vi "PollEngine.Main.vi"(8 "error in (no error)":errorcluster, 11 "Parameters":T1 {"Settings"."Data Refs"."Write Refs" format="%.0x"; "Settings"."Data Refs"."Read Refs" format="%.0x"; "Settings"."Write Locations"."DataType" items=["Boolean"=1, "SByte"=2, "Byte"=3, "Int16"=4, "UInt16"=5, "Int32"=6, "UInt32"=7, "Int64"=8, "UInt64"=9, "Float"=10, "Double"=11, "String"=12, "DateTime"=13, "ByteString"=15, "Array of Boolean"=101, "Array of SByte"=102, "Array of Byte"=103, "Array of Int16"=104, "Array of UInt16"=105, "Array of Int32"=106, "Array of UInt32"=107, "Array of Int64"=108, "Array of UInt64"=109, "Array of Float"=110, "Array of Double"=111, "Array of String"=112, "Array of DateTime"=113, "Array of ByteString"=115]; "Settings"."StatusRefs"."Chan Refs" format="%.0x"}) -> ()   [LabVIEW 2013, in "OPC UA Client Engine.lvlib"]
uses:
  OPC UA Client Engine.lvlib
  Types/PollEngine.Parameters.ctl
  Shared/Compiled.Settings.ctl
  Shared/Connection.Properties.ctl
  Shared/PollEngine.Settings.ctl
  <vilib>/NI Veristand/Custom Device API/Data Reference.ctl
  Shared/WriteData.Info.ctl
  Shared/ReadWriteRefs.ctl
  Stop FG/Stop Global Commands.ctl
  Shared/DataRefs.Location.ctl
  <vilib>/OPCUA/client/Write Bool.vi
  <vilib>/OPCUA/client/Write SByte.vi
  <vilib>/OPCUA/client/Write Byte.vi
  <vilib>/OPCUA/client/Write Int16.vi
  <vilib>/OPCUA/client/Write UInt16.vi
  <vilib>/OPCUA/client/Write Int32.vi
  <vilib>/OPCUA/client/Write UInt32.vi
  <vilib>/OPCUA/client/Write Int64.vi
  <vilib>/OPCUA/client/Write UInt64.vi
  <vilib>/OPCUA/client/Write Float.vi
  <vilib>/OPCUA/client/Write Double.vi
  <vilib>/OPCUA/client/Write DateTime.vi
  <vilib>/OPCUA/client/Write Bool Array.vi
  <vilib>/OPCUA/client/Write SByte Array.vi
  <vilib>/OPCUA/client/Write Byte Array.vi
  <vilib>/OPCUA/client/Write Int16 Array.vi
  <vilib>/OPCUA/client/Write UInt16 Array.vi
  <vilib>/OPCUA/client/Write Int32 Array.vi
  <vilib>/OPCUA/client/Write UInt32 Array.vi
  <vilib>/OPCUA/client/Write Int64 Array.vi
  <vilib>/OPCUA/client/Write UInt64 Array.vi
  <vilib>/OPCUA/client/Write Float Array.vi
  <vilib>/OPCUA/client/Write Double Array.vi
  <vilib>/OPCUA/client/Write DateTime Array.vi
  <vilib>/OPCUA/NI OPC UA Client.lvlib
  Stop FG/Stop FG.lvlib
  Error Handling API/Error Handling API.lvlib
  Shared/OPC UA Client Shared.lvlib
  <vilib>/NI Veristand/Custom Device API/Custom Device API.lvlib
panel:
  in  "Parent":string
  out "Read Code":i32
  out "Write Code":i32
  out "Read Table":variant
  out "Write Table":variant
  out "error out":errorcluster
  in  "stop":bool
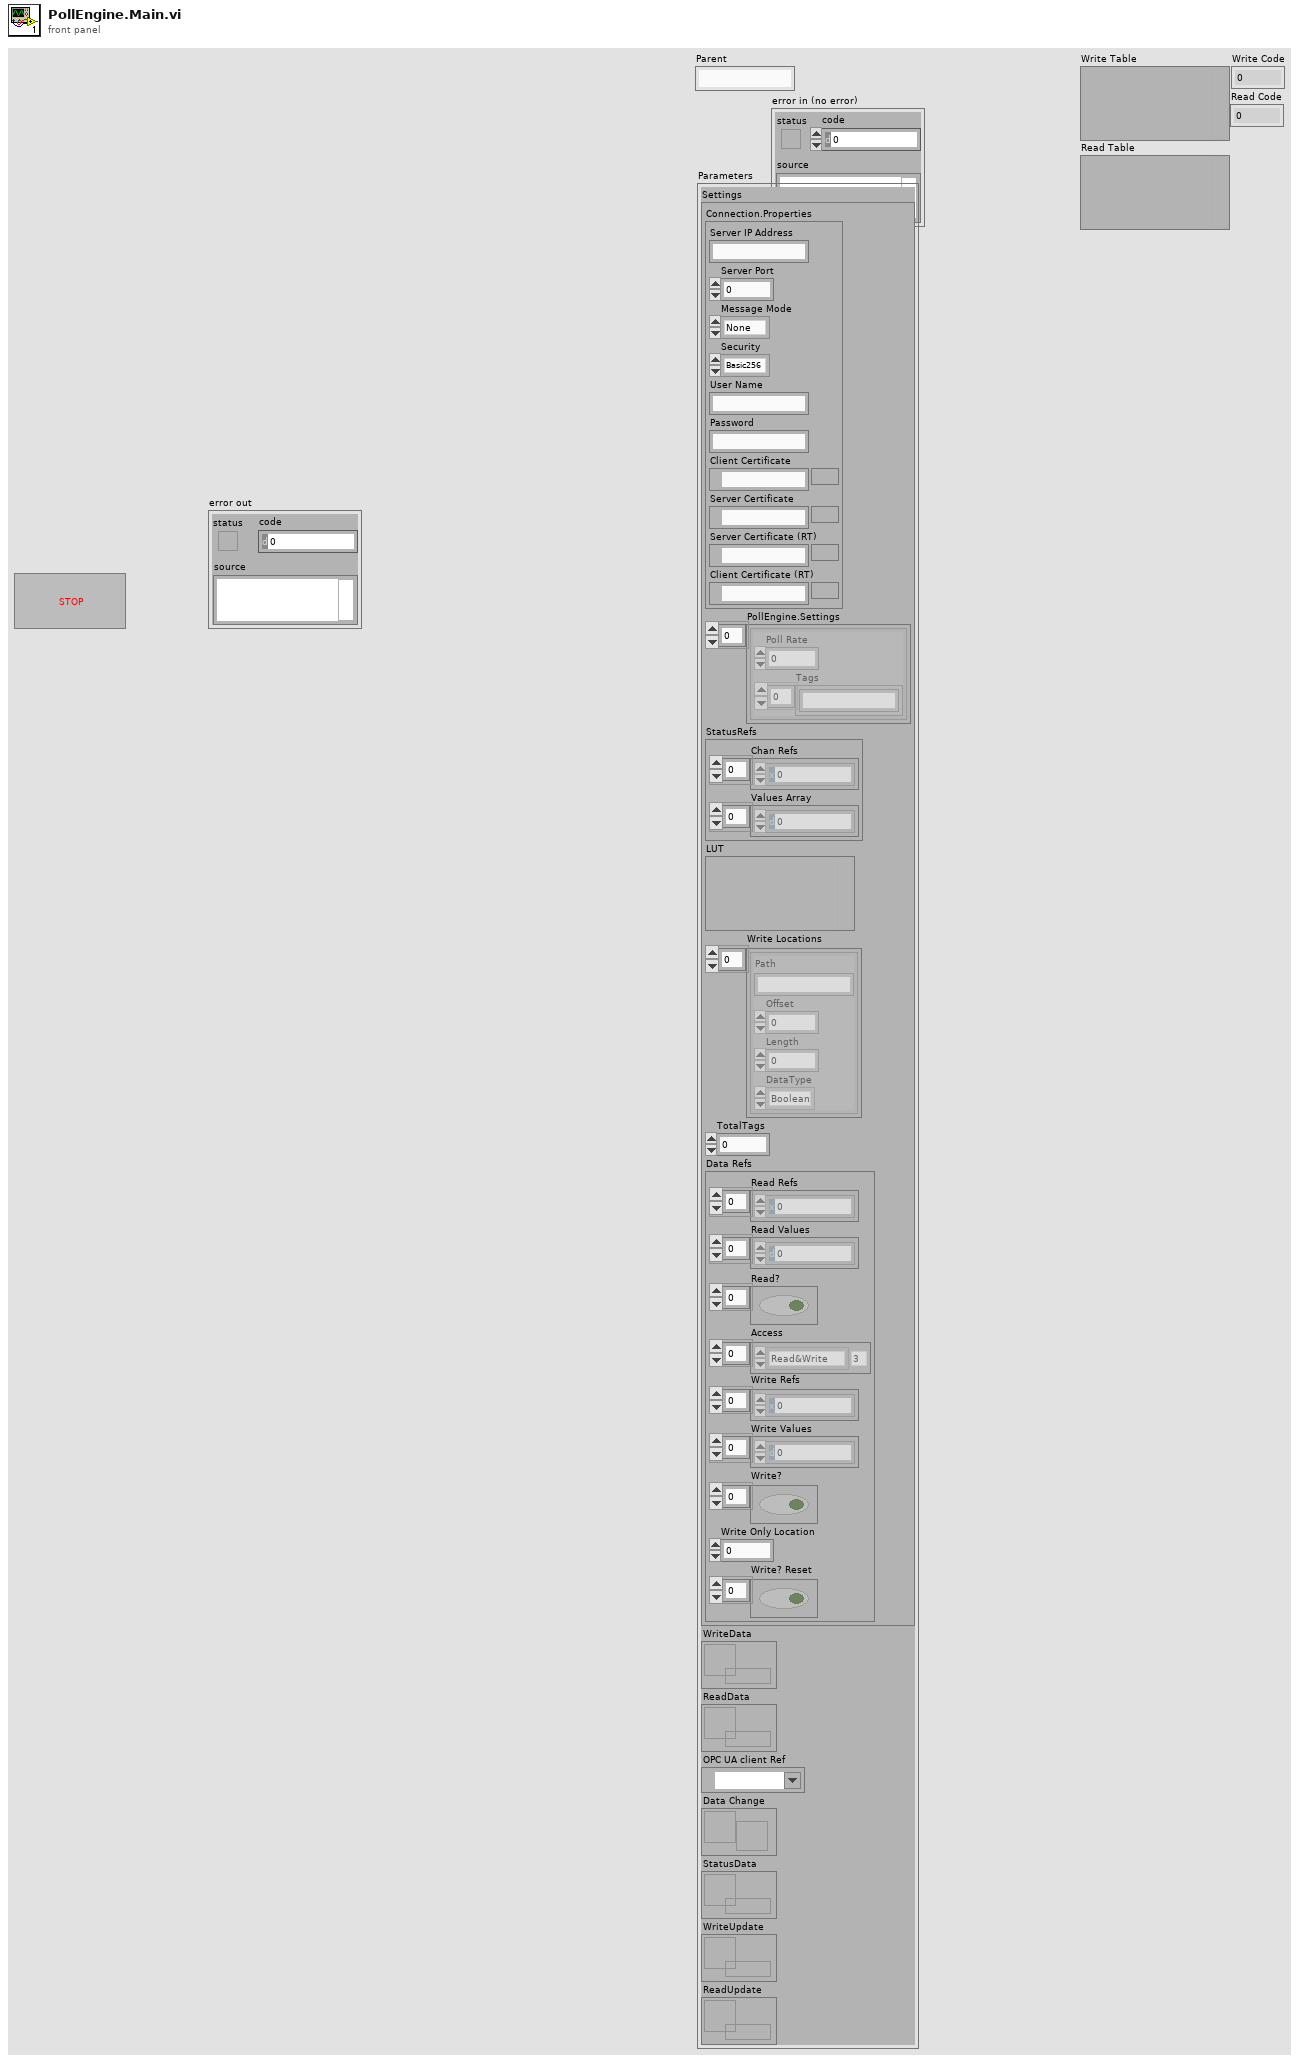
[diagram p1: front panel]
types:
  T1 = typedef "OPC UA Client Engine.lvlib/PollEngine.Parameters.ctl" = cluster{"Settings":T2, "WriteData":refnum<k33>, "ReadData":refnum<k33>, "OPC UA client Ref":refnum<k21>, "Data Change":refnum<user-event>, "StatusData":refnum<k33>, "WriteUpdate":refnum<k33>, "ReadUpdate":refnum<k33>}
  T2 = typedef "OPC UA Client Shared.lvlib/Compiled.Settings.ctl" = cluster{"Connection.Properties":T3, "PollEngine.Settings":T4[], "StatusRefs":cluster{"Chan Refs":T5[], "Values Array":dbl[]}, "LUT":variant, "Write Locations":T6[], "TotalTags":u32, "Data Refs":T7}
  T3 = typedef "OPC UA Client Shared.lvlib/Connection.Properties.ctl" = cluster{"Server IP Address":string, "Server Port":u16, "Message Mode":enum16{"None", "Sign", "Sign and Encrypt"}, "Security":enum16{"Basic256", "Basic128Rsa15"}, "User Name":string, "Password":string, "Client Certificate":path, "Server Certificate":path, "Server Certificate (RT)":path, "Client Certificate (RT)":path}
  T4 = typedef "OPC UA Client Shared.lvlib/PollEngine.Settings.ctl" = cluster{"Poll Rate":dbl, "Tags":string[]}
  T5 = typedef "Custom Device API.lvlib/Data Reference.ctl" = i32
  T6 = typedef "OPC UA Client Shared.lvlib/WriteData.Info.ctl" = cluster{"Path":string, "Offset":i32, "Length":i32, "DataType":u32}
  T7 = typedef "OPC UA Client Shared.lvlib/ReadWriteRefs.ctl" = cluster{"Read Refs":T5[], "Read Values":dbl[], "Read?":bool[], "Access":enum8{"Null", "Read", "Write", "Read&Write"}[], "Write Refs":T5[], "Write Values":dbl[], "Write?":bool[], "Write Only Location":u32, "Write? Reset":bool[]}
  T8 = typedef "OPC UA Client Engine.lvlib/PollEngine.StateVariables.ctl" = cluster{"SubscriptionIDs":u32[], "OPCEvent":refnum<event-registration>, "StopRef":T9, "Parent":string, "ParentVI":refnum<vi>}
  T9 = typedef "OPC UA Client Engine.lvlib/Stop FG.lvlib/Stop Global Ref.ctl" = refnum<vi>
  T10 = typedef "OPC UA Client Engine.lvlib/Stop FG.lvlib/Stop Global Commands.ctl" = enum16{"Write", "Read", "Reset"}
  T11 = typedef "OPC UA Client Shared.lvlib/DataRefs.Location.ctl" = cluster{"Offset":i32, "Length":i32}
  T12 = cluster{"Item URL":string, "Item Value":variant, "Timestamp":timestamp, "DataType":u32, "status code":u32}[]
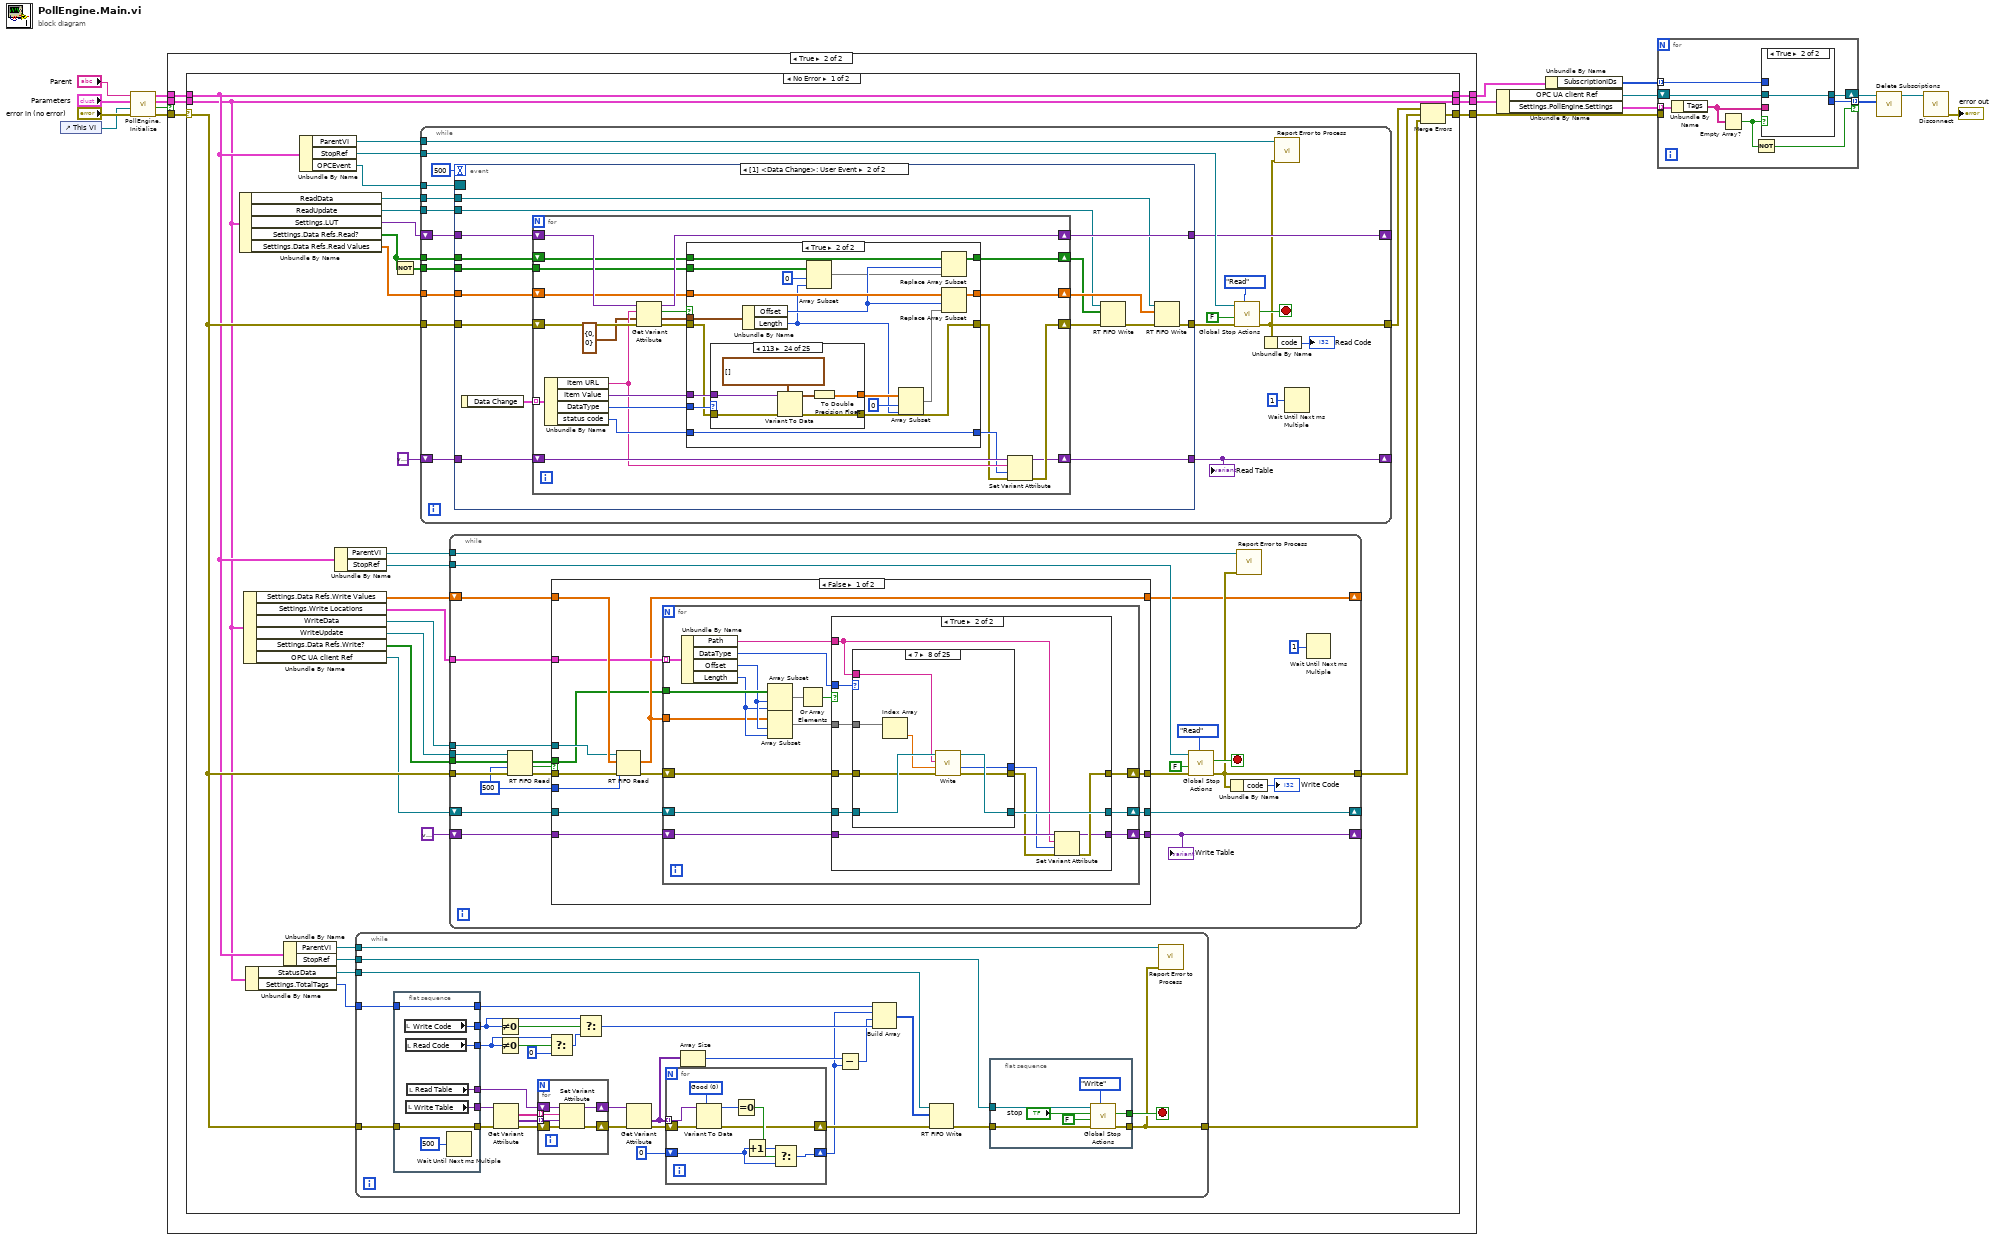
[diagram p0: block diagram]
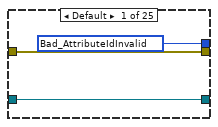
[diagram p4: hidden frame]
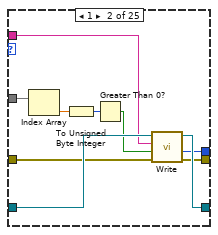
[diagram p5: hidden frame]
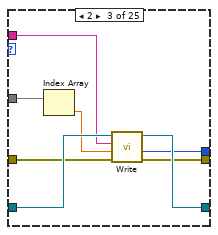
[diagram p6: hidden frame]
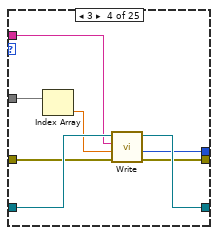
[diagram p7: hidden frame]
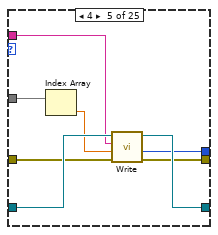
[diagram p8: hidden frame]
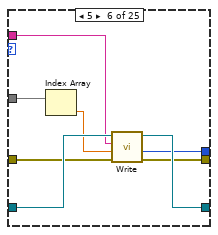
[diagram p9: hidden frame]
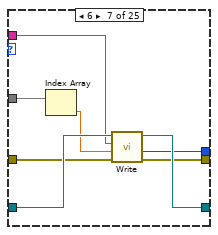
[diagram p10: hidden frame]
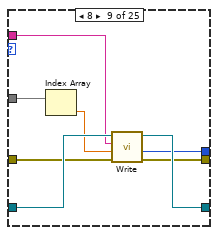
[diagram p11: hidden frame]
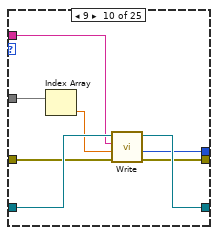
[diagram p12: hidden frame]
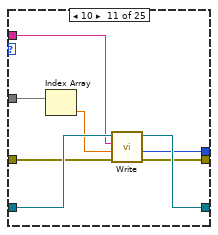
[diagram p13: hidden frame]
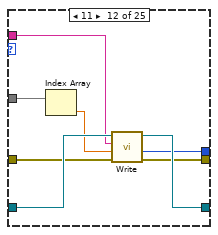
[diagram p14: hidden frame]
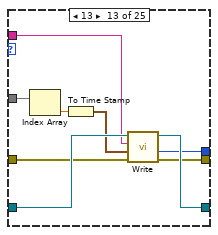
[diagram p15: hidden frame]
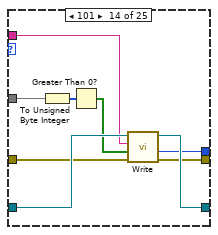
[diagram p16: hidden frame]
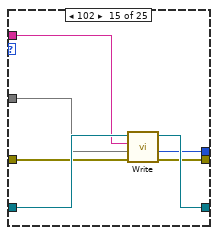
[diagram p17: hidden frame]
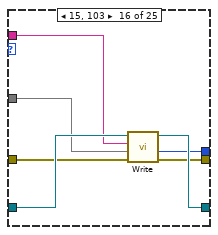
[diagram p18: hidden frame]
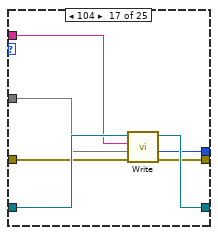
[diagram p19: hidden frame]
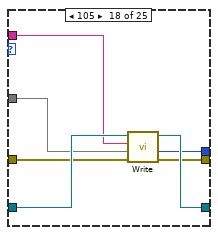
[diagram p20: hidden frame]
diagram:
  n1 = control-ref of="This VI"() -> (w3:refnum<vi>)
  n2 = call "PollEngine.Initialize.vi"("error in (no error)"="error in (no error)", "Parent VI"=w3, "Parameters in"="Parameters", "Parent"="Parent") -> ("error out"=w14:errorcluster, "notification"=w9:bool, "Parameters out"=w10:T1, "Settings"=w8:T8)  [unwired: 4 in]
  n3 = case shown="True" w9 {
    tunnel: w8 -> [w20 w24]
    tunnel: w14 -> [w21 w27]
    tunnel: [w21 w26] -> w13
    tunnel: w10 -> [w19 w25]
    tunnel: [w20 w23] -> w4
    tunnel: [w19 w22] -> w7
    frame False {
    }
    frame True {
      n4 = case shown="No Error" w27 {
        selector: w27 -> [w54 w624]
        tunnel: [w53 w624] -> w26
        tunnel: w25 -> [w39 w623]
        tunnel: w24 -> [w40 w622]
        tunnel: [w40 w622] -> w23
        tunnel: [w39 w623] -> w22
        frame No Error {
          n5 = Unbundle By Name(w39) -> ("ReadData"=w48:refnum<k33>, "ReadUpdate"=w31:refnum<k33>, "Settings.LUT"=w47:variant, "Settings.Data Refs.Read?"=w30:bool[], "Settings.Data Refs.Read Values"=w28:dbl[])
          n6 = Unbundle By Name(w39) -> ("Settings.Data Refs.Write Values"=w52:dbl[], "Settings.Write Locations"=w51:T6[], "WriteData"=w50:refnum<k33>, "WriteUpdate"=w33:refnum<k33>, "Settings.Data Refs.Write?"=w32:bool[], "OPC UA client Ref"=w49:refnum<k21>)
          n7 = Unbundle By Name(w39) -> ("StatusData"=w46:refnum<k33>, "Settings.TotalTags"=w45:u32)
          n8 = Unbundle By Name(w40) -> ("ParentVI"=w36:refnum<vi>, "StopRef"=w41:T9)
          n9 = Unbundle By Name(w40) -> ("ParentVI"=w34:refnum<vi>, "StopRef"=w43:T9, "OPCEvent"=w44:refnum<event-registration>)
          n10 = Unbundle By Name(w40) -> ("ParentVI"=w35:refnum<vi>, "StopRef"=w42:T9)
          n11 = while {
            tunnel: w45 -> [w60]
            tunnel: w54 -> [w79]
            tunnel: w41 -> [w78]
            tunnel: w46 -> [w67]
            tunnel: [w59] -> w38
            tunnel: w36 -> [w58]
            stop <- w77 stop-if-true
            n12 = flat-sequence {
              tunnel: [w112] -> w64
              tunnel: [w111] -> w89
              tunnel: [w110] -> w65
              tunnel: w79 -> [w110]
              tunnel: [w109] -> w75
              tunnel: [w108] -> w73
              tunnel: [w106] -> w61
              tunnel: w60 -> [w106]
              frame #0 {
                n13 = local read "Write Code"() -> (w109:i32)
                n14 = local read "Read Code"() -> (w108:i32)
                n15 = local read "Write Table"() -> (w111:variant)
                n16 = local read "Read Table"() -> (w112:variant)
                n17 = Wait Until Next ms Multiple(millisecond multiple=u32 500) -> ()  [unwired: 1 out]
              }
            }
            n18 = Get Variant Attribute(Variant=w89, error in=w65) -> (names=w88:string[], values=w87:variant[], error out=w86:errorcluster)  [unwired: 2 in, 1 out]
            n19 = Not Equal To 0?(x=w75) -> (x != 0?=w76:bool)
            n20 = Not Equal To 0?(x=w73) -> (x != 0?=w72:bool)
            n21 = for {
              tunnel: w88 -> [w118] mode=indexing
              tunnel: w87 -> [w117] mode=indexing
              shift-right: [w115] -> w85
              shift-left: w64 -> [w116]
              shift-right: [w113] -> w84
              shift-left: w86 -> [w114]
              n22 = Set Variant Attribute(Variant=w116, name=w118, value=w117, error in=w114) -> (Variant out=w115:variant, error out=w113:errorcluster)  [unwired: 1 out]
            }
            n23 = Select(t=w73, s=w72, f=0) -> (s? t:f=w74:i32)
            n24 = Select(t=w75, s=w76, f=w74) -> (s? t:f=w70:i32)
            n25 = Get Variant Attribute(Variant=w85, error in=w84) -> (values=w81:variant[], error out=w83:errorcluster)  [unwired: 2 in, 2 out]
            n26 = for {
              tunnel: w81 -> [w103] mode=indexing
              shift-right: [w98] -> w63
              shift-left: 0 -> [w100]
              shift-right: [w97] -> w69
              shift-left: w83 -> [w105]
              w104 = u32 0 items=["Good"=0, "Bad_AttributeIdInvalid"=2153906176, "Bad_BrowseDirectionInvalid"=2152529920, "Bad_BrowseNameInvalid"=2153775104, "Bad_ContentFilterInvalid"=2152202240, "Bad_ContinuationPointInvalid"=2152333312, "Bad_DataEncodingInvalid"=2151153664, "Bad_DataEncodingUnsupported"=2151219200, "Bad_EventFilterInvalid"=2152136704, "Bad_FilterNotAllowed"=2152005632, "Bad_FilterOperandInvalid"=2160132096, "Bad_HistoryOperationInvalid"=2154889216, "Bad_HistoryOperationUnsupported"=2154954752, "Bad_IndexRangeInvalid"=2151022592, "Bad_IndexRangeNoData"=2151088128, "Bad_MonitoredItemFilterInvalid"=2151874560, "Bad_MonitoredItemFilterUnsupported"=2151940096, "Bad_MonitoredItemIdInvalid"=2151809024, "Bad_MonitoringModeInvalid"=2151743488, "Bad_NoCommunication"=2150694912, "Bad_NoContinuationPoints"=2152398848, "Bad_NodeClassInvalid"=2153709568, "Bad_NodeIdInvalid"=2150825984, "Bad_NodeIdUnknown"=2150891520, "Bad_NoDeleteRights"=2154364928, "Bad_NodeNotInView"=2152595456, "Bad_NotFound"=2151546880, "Bad_NotImplemented"=2151677952, "Bad_NotReadable"=2151284736, "Bad_NotSupported"=2151481344, "Bad_NotWritable"=2151350272, "Bad_ObjectDeleted"=2151612416, "Bad_OutOfRange"=2151415808, "Bad_ReferenceTypeIdInvalid"=2152464384, "Bad_SourceNodeIdInvalid"=2154037248, "Bad_StructureMissing"=2152071168, "Bad_TargetNodeIdInvalid"=2154102784, "Bad_TypeDefinitionInvalid"=2153971712, "Bad_TypeMismatch"=2155085824, "Bad_WaitingForInitialData"=2150760448] ("status")
              n27 = Variant To Data(error in=w105, type=w104, Variant=w103) -> (data=w102:u32, error out=w97:errorcluster)
              n28 = Equal To 0?(x=w102) -> (x = 0?=w101:bool)
              n29 = Increment(x=w100) -> (x+1=w99:i32)
              n30 = Select(t=w99, s=w101, f=w100) -> (s? t:f=w98:i32)
            }
            n31 = Array Size(array=w81) -> (size(s)=w80:i32)
            n32 = Subtract(x=w80, y=w63) -> (x-y=w62:i32)
            n33 = Build Array(w61, w63, w62, w70) -> (w66:u32[])
            n34 = RT FIFO Write(0:w67, 1:w66, 3:w69) -> (11:w68:errorcluster)  [unwired: 2 in, 3 out]
            n35 = flat-sequence {
              tunnel: w78 -> [w94]
              tunnel: [w93] -> w77
              tunnel: w68 -> [w92]
              tunnel: [w91] -> w59
              frame #0 {
                n36 = call "Global Stop Actions.vi"("Command"=Stop_Global_Commands."Write", "error in (no error)"=w92, "Stop on Error?"=FALSE, "Stop?"="stop", "vi reference"=w94) -> ("error out"=w91:errorcluster, "Latched Stop"=w93:bool)  [unwired: 4 in, 1 out]
              }
            }
            n37 = call "Report Error to Process.vi"("Error"=w59, "This VI"=w58) -> ()  [unwired: 10 in]
          }
          n38 = Not(x=w30) -> (.not. x?=w29:bool[])
          n39 = while {
            tunnel: w44 -> [w399]
            shift-right: [w389] -> _
            shift-left: w47 -> [w396]
            tunnel: w48 -> [w383]
            tunnel: w54 -> [w397]
            tunnel: [w385] -> w37
            shift-right: [w387] -> _
            shift-left: variant ("variant") -> [w395]
            tunnel: w43 -> [w390]
            tunnel: w34 -> [w384]
            tunnel: w31 -> [w382]
            tunnel: w30 -> [w381]
            tunnel: w29 -> [w380]
            tunnel: w28 -> [w379]
            stop <- w391 stop-if-true
            n40 = event shown="[1] <Data Change>: User Event" {
              selector: w399 -> [_ _]
              dyn-events: _ -> [_ _]
              timeout: 500 -> [_ _]
              tunnel: w397 -> [w402 w415]
              tunnel: [w402 w411] -> w393
              tunnel: w396 -> [w401 w417]
              tunnel: [w401 w416] -> w389
              tunnel: w395 -> [w400 w414]
              tunnel: [w400 w413] -> w387
              tunnel: w379 -> [_ w412]
              tunnel: w383 -> [_ w409]
              tunnel: w382 -> [_ w406]
              tunnel: w381 -> [_ w404]
              tunnel: w380 -> [_ w403]
              event Timeout {
                n41 = event-data() -> ()  [unwired: 1 in, 2 out]
              }
              event User Event {
                n42 = event-data() -> ("Data Change"=w418:T12)  [unwired: 1 in]
                n43 = for {
                  tunnel: w418 -> [w440] mode=indexing
                  shift-right: [w436] -> w416
                  shift-left: w417 -> [w438]
                  shift-right: [w426] -> w408
                  shift-left: w415 -> [w435]
                  shift-right: [w425] -> w413
                  shift-left: w414 -> [w430]
                  shift-right: [w422] -> w410
                  shift-left: w412 -> [w423]
                  shift-right: [w420] -> w405
                  shift-left: w404 -> [w421]
                  tunnel: w403 -> [w419]
                  n44 = Unbundle By Name(w440) -> ("Item URL"=w429:string, "Item Value"=w439:variant, "DataType"=w434:u32, "status code"=w432:u32)
                  n45 = Get Variant Attribute(Variant=w438, name=w429, default value (empty Variant)=T11 {"Offset"=0, "Length"=0} ("cluster"), error in=w435) -> (duplicate Variant=w436:variant, found=w431:bool, value=w437:T11, error out=w433:errorcluster)
                  n46 = case shown="True" w431 {
                    tunnel: w439 -> [_ w462]
                    tunnel: w437 -> [_ w457]
                    tunnel: [w444 w456] -> w427
                    tunnel: w434 -> [_ w461]
                    tunnel: w433 -> [w444 w460]
                    tunnel: w432 -> [_ w459]
                    tunnel: [w443 w459] -> w428
                    tunnel: w423 -> [w442 w458]
                    tunnel: [w442 w453] -> w422
                    tunnel: w421 -> [w441 w449]
                    tunnel: [w441 w450] -> w420
                    tunnel: w419 -> [_ w446]
                    frame False {
                      w443 = u32 2153906176 items=["Good"=0, "Bad_AttributeIdInvalid"=2153906176, "Bad_BrowseDirectionInvalid"=2152529920, "Bad_BrowseNameInvalid"=2153775104, "Bad_ContentFilterInvalid"=2152202240, "Bad_ContinuationPointInvalid"=2152333312, "Bad_DataEncodingInvalid"=2151153664, "Bad_DataEncodingUnsupported"=2151219200, "Bad_EventFilterInvalid"=2152136704, "Bad_FilterNotAllowed"=2152005632, "Bad_FilterOperandInvalid"=2160132096, "Bad_HistoryOperationInvalid"=2154889216, "Bad_HistoryOperationUnsupported"=2154954752, "Bad_IndexRangeInvalid"=2151022592, "Bad_IndexRangeNoData"=2151088128, "Bad_MonitoredItemFilterInvalid"=2151874560, "Bad_MonitoredItemFilterUnsupported"=2151940096, "Bad_MonitoredItemIdInvalid"=2151809024, "Bad_MonitoringModeInvalid"=2151743488, "Bad_NoCommunication"=2150694912, "Bad_NoContinuationPoints"=2152398848, "Bad_NodeClassInvalid"=2153709568, "Bad_NodeIdInvalid"=2150825984, "Bad_NodeIdUnknown"=2150891520, "Bad_NoDeleteRights"=2154364928, "Bad_NodeNotInView"=2152595456, "Bad_NotFound"=2151546880, "Bad_NotImplemented"=2151677952, "Bad_NotReadable"=2151284736, "Bad_NotSupported"=2151481344, "Bad_NotWritable"=2151350272, "Bad_ObjectDeleted"=2151612416, "Bad_OutOfRange"=2151415808, "Bad_ReferenceTypeIdInvalid"=2152464384, "Bad_SourceNodeIdInvalid"=2154037248, "Bad_StructureMissing"=2152071168, "Bad_TargetNodeIdInvalid"=2154102784, "Bad_TypeDefinitionInvalid"=2153971712, "Bad_TypeMismatch"=2155085824, "Bad_WaitingForInitialData"=2150760448] ("status")
                    }
                    frame True {
                      n47 = case shown="113" w461 {
                        tunnel: w462 -> [w470 w477 w484 w491 w498 w505 w512 w519 w526 w533 w540 w547 w554 w560 w566 w572 w578 w584 w590 w596 w602 w608 w614 w620 _]
                        tunnel: w460 -> [w469 w476 w483 w490 w497 w504 w511 w518 w525 w532 w539 w546 w553 w559 w565 w571 w577 w583 w589 w595 w601 w607 w613 w619 w621]
                        tunnel: [w468 w475 w482 w489 w496 w503 w510 w517 w524 w531 w538 w545 w552 w558 w564 w570 w576 w582 w588 w594 w600 w606 w612 w618 w621] -> w456
                        tunnel: [w463 w472 w479 w486 w493 w500 w507 w514 w521 w528 w535 w542 w548 w556 w562 w568 w574 w580 w586 w592 w598 w604 w610 w616 _] -> w455
                        frame 1 {
                          n48 = Variant To Data(error in=w469, type=FALSE, Variant=w470) -> (data=w466:bool, error out=w468:errorcluster)
                          n49 = Boolean To (0,1)(Boolean=w466) -> (0, 1=w465:i16)
                          n50 = To Double Precision Float(number=w465) -> (double precision float=w464:dbl)
                          n51 = Build Array(w464) -> (w463:dbl[])
                        }
                        frame 2 {
                          n52 = Variant To Data(error in=w476, type=i8 0, Variant=w477) -> (data=w471:i8, error out=w475:errorcluster)
                          n53 = To Double Precision Float(number=w471) -> (double precision float=w473:dbl)
                          n54 = Build Array(w473) -> (w472:dbl[])
                        }
                        frame 3 {
                          n55 = Variant To Data(error in=w483, type=u8 0, Variant=w484) -> (data=w478:u8, error out=w482:errorcluster)
                          n56 = To Double Precision Float(number=w478) -> (double precision float=w480:dbl)
                          n57 = Build Array(w480) -> (w479:dbl[])
                        }
                        frame 4 {
                          n58 = Variant To Data(error in=w490, type=i16 0, Variant=w491) -> (data=w485:i16, error out=w489:errorcluster)
                          n59 = To Double Precision Float(number=w485) -> (double precision float=w487:dbl)
                          n60 = Build Array(w487) -> (w486:dbl[])
                        }
                        frame 5 {
                          n61 = Variant To Data(error in=w497, type=u16 0, Variant=w498) -> (data=w492:u16, error out=w496:errorcluster)
                          n62 = To Double Precision Float(number=w492) -> (double precision float=w494:dbl)
                          n63 = Build Array(w494) -> (w493:dbl[])
                        }
                        frame 6 {
                          n64 = Variant To Data(error in=w504, type=0, Variant=w505) -> (data=w499:i32, error out=w503:errorcluster)
                          n65 = To Double Precision Float(number=w499) -> (double precision float=w501:dbl)
                          n66 = Build Array(w501) -> (w500:dbl[])
                        }
                        frame 7 {
                          n67 = Variant To Data(error in=w511, type=u32 0, Variant=w512) -> (data=w506:u32, error out=w510:errorcluster)
                          n68 = To Double Precision Float(number=w506) -> (double precision float=w508:dbl)
                          n69 = Build Array(w508) -> (w507:dbl[])
                        }
                        frame 8 {
                          n70 = Variant To Data(error in=w518, type=i64 0, Variant=w519) -> (data=w513:i64, error out=w517:errorcluster)
                          n71 = To Double Precision Float(number=w513) -> (double precision float=w515:dbl)
                          n72 = Build Array(w515) -> (w514:dbl[])
                        }
                        frame 9 {
                          n73 = Variant To Data(error in=w525, type=u64 0, Variant=w526) -> (data=w520:u64, error out=w524:errorcluster)
                          n74 = To Double Precision Float(number=w520) -> (double precision float=w522:dbl)
                          n75 = Build Array(w522) -> (w521:dbl[])
                        }
                        frame 10 {
                          n76 = Variant To Data(error in=w532, type=sgl 0.0, Variant=w533) -> (data=w527:sgl, error out=w531:errorcluster)
                          n77 = To Double Precision Float(number=w527) -> (double precision float=w529:dbl)
                          n78 = Build Array(w529) -> (w528:dbl[])
                        }
                        frame 11 {
                          n79 = Variant To Data(error in=w539, type=0.0, Variant=w540) -> (data=w534:dbl, error out=w538:errorcluster)
                          n80 = To Double Precision Float(number=w534) -> (double precision float=w536:dbl)
                          n81 = Build Array(w536) -> (w535:dbl[])
                        }
                        frame 13 {
                          n82 = Variant To Data(error in=w546, type=timestamp(0 s since 1904-01-01), Variant=w547) -> (data=w541:timestamp, error out=w545:errorcluster)
                          n83 = To Double Precision Float(number=w541) -> (double precision float=w543:dbl)
                          n84 = Build Array(w543) -> (w542:dbl[])
                        }
                        frame 101 {
                          n85 = Variant To Data(error in=w553, type=bool[] [], Variant=w554) -> (data=w551:bool[], error out=w552:errorcluster)
                          n86 = Boolean To (0,1)(Boolean=w551) -> (0, 1=w550:i16[])
                          n87 = To Double Precision Float(number=w550) -> (double precision float=w548:dbl[])
                        }
                        frame 102 {
                          n88 = Variant To Data(error in=w559, type=i8[] [], Variant=w560) -> (data=w555:i8[], error out=w558:errorcluster)
                          n89 = To Double Precision Float(number=w555) -> (double precision float=w556:dbl[])
                        }
                        frame 15, 103 {
                          n90 = Variant To Data(error in=w565, type=u8[] [], Variant=w566) -> (data=w561:u8[], error out=w564:errorcluster)
                          n91 = To Double Precision Float(number=w561) -> (double precision float=w562:dbl[])
                        }
                        frame 104 {
                          n92 = Variant To Data(error in=w571, type=i16[] [], Variant=w572) -> (data=w567:i16[], error out=w570:errorcluster)
                          n93 = To Double Precision Float(number=w567) -> (double precision float=w568:dbl[])
                        }
                        frame 105 {
                          n94 = Variant To Data(error in=w577, type=u16[] [], Variant=w578) -> (data=w573:u16[], error out=w576:errorcluster)
                          n95 = To Double Precision Float(number=w573) -> (double precision float=w574:dbl[])
                        }
                        frame 106 {
                          n96 = Variant To Data(error in=w583, type=i32[] [], Variant=w584) -> (data=w579:i32[], error out=w582:errorcluster)
                          n97 = To Double Precision Float(number=w579) -> (double precision float=w580:dbl[])
                        }
                        frame 107 {
                          n98 = Variant To Data(error in=w589, type=u32[] [], Variant=w590) -> (data=w585:u32[], error out=w588:errorcluster)
                          n99 = To Double Precision Float(number=w585) -> (double precision float=w586:dbl[])
                        }
                        frame 108 {
                          n100 = Variant To Data(error in=w595, type=i64[] [], Variant=w596) -> (data=w591:i64[], error out=w594:errorcluster)
                          n101 = To Double Precision Float(number=w591) -> (double precision float=w592:dbl[])
                        }
                        frame 109 {
                          n102 = Variant To Data(error in=w601, type=u64[] [], Variant=w602) -> (data=w597:u64[], error out=w600:errorcluster)
                          n103 = To Double Precision Float(number=w597) -> (double precision float=w598:dbl[])
                        }
                        frame 110 {
                          n104 = Variant To Data(error in=w607, type=sgl[] [], Variant=w608) -> (data=w603:sgl[], error out=w606:errorcluster)
                          n105 = To Double Precision Float(number=w603) -> (double precision float=w604:dbl[])
                        }
                        frame 111 {
                          n106 = Variant To Data(error in=w613, type=dbl[] [], Variant=w614) -> (data=w609:dbl[], error out=w612:errorcluster)
                          n107 = To Double Precision Float(number=w609) -> (double precision float=w610:dbl[])
                        }
                        frame 113 {
                          n108 = Variant To Data(error in=w619, type=timestamp[] [], Variant=w620) -> (data=w615:timestamp[], error out=w618:errorcluster)
                          n109 = To Double Precision Float(number=w615) -> (double precision float=w616:dbl[])
                        }
                        frame Default {
                        }
                      }
                      n110 = Unbundle By Name(w457) -> ("Offset"=w452:i32, "Length"=w448:i32)
                      n111 = Array Subset(array=w446, index=0, length=w448) -> (w445:bool[])
                      n112 = Array Subset(array=w455, index=0, length=w448) -> (w454:dbl[])
                      n113 = Replace Array Subset(array=w449, new element=w445, index=w452) -> (w450:bool[])
                      n114 = Replace Array Subset(array=w458, new element=w454, index=w452) -> (w453:dbl[])
                    }
                  }
                  n115 = Set Variant Attribute(Variant=w430, name=w429, value=w428, error in=w427) -> (Variant out=w425:variant, error out=w426:errorcluster)  [unwired: 1 out]
                }
                n116 = RT FIFO Write(0:w406, 1:w405, 3:w408) -> (11:w407:errorcluster)  [unwired: 2 in, 3 out]
                n117 = RT FIFO Write(0:w409, 1:w410, 3:w407) -> (11:w411:errorcluster)  [unwired: 2 in, 3 out]
              }
            }
            "Read Table" <- w387
            n118 = call "Global Stop Actions.vi"("Command"=Stop_Global_Commands."Read", "error in (no error)"=w393, "Stop on Error?"=FALSE, "vi reference"=w390) -> ("error out"=w385:errorcluster, "Latched Stop"=w391:bool)  [unwired: 5 in, 1 out]
            n119 = Unbundle By Name(w385) -> ("code"=→"Read Code":i32)
            n120 = call "Report Error to Process.vi"("Error"=w385, "This VI"=w384) -> ()  [unwired: 10 in]
            n121 = Wait Until Next ms Multiple(millisecond multiple=u32 1) -> ()  [unwired: 1 out]
          }
          n122 = while {
            tunnel: w51 -> [w141]
            shift-right: [w127] -> _
            shift-left: w52 -> [w142]
            tunnel: w50 -> [w139]
            tunnel: w54 -> [w126]
            tunnel: [w128] -> w55
            shift-right: [w138] -> _
            shift-left: w49 -> [w140]
            shift-right: [w137] -> _
            shift-left: variant ("variant") -> [w136]
            tunnel: w42 -> [w132]
            tunnel: w35 -> [w129]
            tunnel: w33 -> [w124]
            tunnel: w32 -> [w123]
            stop <- w133 stop-if-true
            w122 = 500 ("timeout in ms (0)")
            n123 = RT FIFO Read(0:w124, 1:w123, 2:w122, 3:w126) -> (9:w121:bool[], 10:w120:bool, 11:w125:errorcluster)  [unwired: 2 out]
            n124 = case shown="False" w120 {
              tunnel: w142 -> [w154 w378]
              tunnel: w141 -> [w153 _]
              tunnel: w140 -> [w152 w375]
              tunnel: w139 -> [w151 _]
              tunnel: [w150 w375] -> w138
              tunnel: [w149 w376] -> w137
              tunnel: w136 -> [w148 w376]
              tunnel: [w147 w377] -> w134
              tunnel: [w146 w378] -> w127
              tunnel: w125 -> [w145 w377]
              tunnel: w122 -> [w144 _]
              tunnel: w121 -> [w143 _]
              frame False {
                n125 = RT FIFO Read(0:w151, 1:w154, 2:w144, 3:w145) -> (9:w146:dbl[], 11:w155:errorcluster)  [unwired: 3 out]
                n126 = for {
                  tunnel: w143 -> [w167]
                  tunnel: w153 -> [w165] mode=indexing
                  shift-right: [w169] -> w147
                  shift-left: w155 -> [w168]
                  shift-right: [w170] -> w150
                  shift-left: w152 -> [w171]
                  tunnel: w146 -> [w161]
                  shift-right: [w159] -> w149
                  shift-left: w148 -> [w160]
                  n127 = Unbundle By Name(w165) -> ("Path"=w158:string, "DataType"=w162:u32, "Offset"=w164:i32, "Length"=w163:i32)
                  n128 = Array Subset(array=w167, index=w164, length=w163) -> (w156:bool[])
                  n129 = Array Subset(array=w161, index=w164, length=w163) -> (w166:dbl[])
                  n130 = Or Array Elements(Boolean array=w156) -> (logical OR=w157:bool)
                  n131 = case shown="True" w157 {
                    tunnel: w171 -> [w173 w185]
                    tunnel: [w173 w184] -> w170
                    tunnel: [w174 w177] -> w169
                    tunnel: w168 -> [w174 w183]
                    tunnel: w158 -> [_ w175]
                    tunnel: w166 -> [_ w182]
                    tunnel: w162 -> [_ w181]
                    tunnel: w160 -> [w172 w180]
                    tunnel: [w172 w176] -> w159
                    frame False {
                    }
                    frame True {
                      n132 = case shown="7" w181 {
                        tunnel: w185 -> [w188 w198 w206 w214 w222 w230 w238 w246 w254 w262 w270 w278 w287 w296 w303 w310 w317 w324 w331 w338 w345 w352 w359 w366 w374]
                        tunnel: [w188 w197 w205 w213 w221 w229 w237 w245 w253 w261 w269 w277 w286 w295 w302 w309 w316 w323 w330 w337 w344 w351 w358 w365 w373] -> w184
                        tunnel: [w187 w196 w204 w212 w220 w228 w236 w244 w252 w260 w268 w276 w285 w294 w301 w308 w315 w322 w329 w336 w343 w350 w357 w364 w372] -> w178
                        tunnel: w183 -> [w187 w195 w203 w211 w219 w227 w235 w243 w251 w259 w267 w275 w284 w293 w300 w307 w314 w321 w328 w335 w342 w349 w356 w363 w371]
                        tunnel: w182 -> [_ w193 w201 w209 w217 w225 w233 w241 w249 w257 w265 w273 w282 w291 w299 w306 w313 w320 w327 w334 w341 w348 w355 w362 w370]
                        tunnel: w175 -> [_ w190 w200 w208 w216 w224 w232 w240 w248 w256 w264 w272 w280 w289 w298 w305 w312 w319 w326 w333 w340 w347 w354 w361 w369]
                        tunnel: [w186 w189 w199 w207 w215 w223 w231 w239 w247 w255 w263 w271 w279 w288 w297 w304 w311 w318 w325 w332 w339 w346 w353 w360 w367] -> w179
                        frame Default {
                          w186 = u32 2153906176 items=["Good"=0, "Bad_AttributeIdInvalid"=2153906176, "Bad_BrowseDirectionInvalid"=2152529920, "Bad_BrowseNameInvalid"=2153775104, "Bad_ContentFilterInvalid"=2152202240, "Bad_ContinuationPointInvalid"=2152333312, "Bad_DataEncodingInvalid"=2151153664, "Bad_DataEncodingUnsupported"=2151219200, "Bad_EventFilterInvalid"=2152136704, "Bad_FilterNotAllowed"=2152005632, "Bad_FilterOperandInvalid"=2160132096, "Bad_HistoryOperationInvalid"=2154889216, "Bad_HistoryOperationUnsupported"=2154954752, "Bad_IndexRangeInvalid"=2151022592, "Bad_IndexRangeNoData"=2151088128, "Bad_MonitoredItemFilterInvalid"=2151874560, "Bad_MonitoredItemFilterUnsupported"=2151940096, "Bad_MonitoredItemIdInvalid"=2151809024, "Bad_MonitoringModeInvalid"=2151743488, "Bad_NoCommunication"=2150694912, "Bad_NoContinuationPoints"=2152398848, "Bad_NodeClassInvalid"=2153709568, "Bad_NodeIdInvalid"=2150825984, "Bad_NodeIdUnknown"=2150891520, "Bad_NoDeleteRights"=2154364928, "Bad_NodeNotInView"=2152595456, "Bad_NotFound"=2151546880, "Bad_NotImplemented"=2151677952, "Bad_NotReadable"=2151284736, "Bad_NotSupported"=2151481344, "Bad_NotWritable"=2151350272, "Bad_ObjectDeleted"=2151612416, "Bad_OutOfRange"=2151415808, "Bad_ReferenceTypeIdInvalid"=2152464384, "Bad_SourceNodeIdInvalid"=2154037248, "Bad_StructureMissing"=2152071168, "Bad_TargetNodeIdInvalid"=2154102784, "Bad_TypeDefinitionInvalid"=2153971712, "Bad_TypeMismatch"=2155085824, "Bad_WaitingForInitialData"=2150760448] ("status")
                        }
                        frame 1 {
                          n133 = Index Array(array=w193) -> (element=w194:dbl)  [unwired: 1 in]
                          n134 = To Unsigned Byte Integer(number=w194) -> (unsigned 8bit integer=w191:u8)
                          n135 = Greater Than 0?(x=w191) -> (x > 0?=w192:bool)
                          n136 = call-poly <vilib>:"Write.vi"("error in (no error)"=w195, "value"=w192, "node path"=w190, "OPC UA client refnum in"=w198) -> ("error out"=w196:errorcluster, "status"=w189:u32, "OPC UA client refnum out"=w197:refnum<k21>)  [unwired: 5 in]
                        }
                        frame 2 {
                          n137 = Index Array(array=w201) -> (element=w202:dbl)  [unwired: 1 in]
                          n138 = call-poly <vilib>:"Write.vi"("error in (no error)"=w203, "value"=w202, "node path"=w200, "OPC UA client refnum in"=w206) -> ("error out"=w204:errorcluster, "status"=w199:u32, "OPC UA client refnum out"=w205:refnum<k21>)  [unwired: 5 in]
                        }
                        frame 3 {
                          n139 = Index Array(array=w209) -> (element=w210:dbl)  [unwired: 1 in]
                          n140 = call-poly <vilib>:"Write.vi"("error in (no error)"=w211, "value"=w210, "node path"=w208, "OPC UA client refnum in"=w214) -> ("error out"=w212:errorcluster, "status"=w207:u32, "OPC UA client refnum out"=w213:refnum<k21>)  [unwired: 5 in]
                        }
                        frame 4 {
                          n141 = Index Array(array=w217) -> (element=w218:dbl)  [unwired: 1 in]
                          n142 = call-poly <vilib>:"Write.vi"("error in (no error)"=w219, "value"=w218, "node path"=w216, "OPC UA client refnum in"=w222) -> ("error out"=w220:errorcluster, "status"=w215:u32, "OPC UA client refnum out"=w221:refnum<k21>)  [unwired: 5 in]
                        }
                        frame 5 {
                          n143 = Index Array(array=w225) -> (element=w226:dbl)  [unwired: 1 in]
                          n144 = call-poly <vilib>:"Write.vi"("error in (no error)"=w227, "value"=w226, "node path"=w224, "OPC UA client refnum in"=w230) -> ("error out"=w228:errorcluster, "status"=w223:u32, "OPC UA client refnum out"=w229:refnum<k21>)  [unwired: 5 in]
                        }
                        frame 6 {
                          n145 = Index Array(array=w233) -> (element=w234:dbl)  [unwired: 1 in]
                          n146 = call-poly <vilib>:"Write.vi"("error in (no error)"=w235, "value"=w234, "node path"=w232, "OPC UA client refnum in"=w238) -> ("error out"=w236:errorcluster, "status"=w231:u32, "OPC UA client refnum out"=w237:refnum<k21>)  [unwired: 5 in]
                        }
                        frame 7 {
                          n147 = Index Array(array=w241) -> (element=w242:dbl)  [unwired: 1 in]
                          n148 = call-poly <vilib>:"Write.vi"("error in (no error)"=w243, "value"=w242, "node path"=w240, "OPC UA client refnum in"=w246) -> ("error out"=w244:errorcluster, "status"=w239:u32, "OPC UA client refnum out"=w245:refnum<k21>)  [unwired: 5 in]
                        }
                        frame 8 {
                          n149 = Index Array(array=w249) -> (element=w250:dbl)  [unwired: 1 in]
                          n150 = call-poly <vilib>:"Write.vi"("error in (no error)"=w251, "value"=w250, "node path"=w248, "OPC UA client refnum in"=w254) -> ("error out"=w252:errorcluster, "status"=w247:u32, "OPC UA client refnum out"=w253:refnum<k21>)  [unwired: 5 in]
                        }
                        frame 9 {
                          n151 = Index Array(array=w257) -> (element=w258:dbl)  [unwired: 1 in]
                          n152 = call-poly <vilib>:"Write.vi"("error in (no error)"=w259, "value"=w258, "node path"=w256, "OPC UA client refnum in"=w262) -> ("error out"=w260:errorcluster, "status"=w255:u32, "OPC UA client refnum out"=w261:refnum<k21>)  [unwired: 5 in]
                        }
                        frame 10 {
                          n153 = Index Array(array=w265) -> (element=w266:dbl)  [unwired: 1 in]
                          n154 = call-poly <vilib>:"Write.vi"("error in (no error)"=w267, "value"=w266, "node path"=w264, "OPC UA client refnum in"=w270) -> ("error out"=w268:errorcluster, "status"=w263:u32, "OPC UA client refnum out"=w269:refnum<k21>)  [unwired: 5 in]
                        }
                        frame 11 {
                          n155 = Index Array(array=w273) -> (element=w274:dbl)  [unwired: 1 in]
                          n156 = call-poly <vilib>:"Write.vi"("error in (no error)"=w275, "value"=w274, "node path"=w272, "OPC UA client refnum in"=w278) -> ("error out"=w276:errorcluster, "status"=w271:u32, "OPC UA client refnum out"=w277:refnum<k21>)  [unwired: 5 in]
                        }
                        frame 13 {
                          n157 = Index Array(array=w282) -> (element=w283:dbl)  [unwired: 1 in]
                          n158 = To Time Stamp(1:w283) -> (0:w281:timestamp)
                          n159 = call-poly <vilib>:"Write.vi"("error in (no error)"=w284, "value"=w281, "node path"=w280, "OPC UA client refnum in"=w287) -> ("error out"=w285:errorcluster, "status"=w279:u32, "OPC UA client refnum out"=w286:refnum<k21>)  [unwired: 5 in]
                        }
                        frame 101 {
                          n160 = To Unsigned Byte Integer(number=w291) -> (unsigned 8bit integer=w292:u8[])
                          n161 = Greater Than 0?(x=w292) -> (x > 0?=w290:bool[])
                          n162 = call-poly <vilib>:"Write.vi"("error in (no error)"=w293, "value"=w290, "node path"=w289, "OPC UA client refnum in"=w296) -> ("error out"=w294:errorcluster, "status"=w288:u32, "OPC UA client refnum out"=w295:refnum<k21>)  [unwired: 5 in]
                        }
                        frame 102 {
                          n163 = call-poly <vilib>:"Write.vi"("error in (no error)"=w300, "value"=w299, "node path"=w298, "OPC UA client refnum in"=w303) -> ("error out"=w301:errorcluster, "status"=w297:u32, "OPC UA client refnum out"=w302:refnum<k21>)  [unwired: 5 in]
                        }
                        frame 15, 103 {
                          n164 = call-poly <vilib>:"Write.vi"("error in (no error)"=w307, "value"=w306, "node path"=w305, "OPC UA client refnum in"=w310) -> ("error out"=w308:errorcluster, "status"=w304:u32, "OPC UA client refnum out"=w309:refnum<k21>)  [unwired: 5 in]
                        }
                        frame 104 {
                          n165 = call-poly <vilib>:"Write.vi"("error in (no error)"=w314, "value"=w313, "node path"=w312, "OPC UA client refnum in"=w317) -> ("error out"=w315:errorcluster, "status"=w311:u32, "OPC UA client refnum out"=w316:refnum<k21>)  [unwired: 5 in]
                        }
                        frame 105 {
                          n166 = call-poly <vilib>:"Write.vi"("error in (no error)"=w321, "value"=w320, "node path"=w319, "OPC UA client refnum in"=w324) -> ("error out"=w322:errorcluster, "status"=w318:u32, "OPC UA client refnum out"=w323:refnum<k21>)  [unwired: 5 in]
                        }
                        frame 106 {
                          n167 = call-poly <vilib>:"Write.vi"("error in (no error)"=w328, "value"=w327, "node path"=w326, "OPC UA client refnum in"=w331) -> ("error out"=w329:errorcluster, "status"=w325:u32, "OPC UA client refnum out"=w330:refnum<k21>)  [unwired: 5 in]
                        }
                        frame 107 {
                          n168 = call-poly <vilib>:"Write.vi"("error in (no error)"=w335, "value"=w334, "node path"=w333, "OPC UA client refnum in"=w338) -> ("error out"=w336:errorcluster, "status"=w332:u32, "OPC UA client refnum out"=w337:refnum<k21>)  [unwired: 5 in]
                        }
                        frame 108 {
                          n169 = call-poly <vilib>:"Write.vi"("error in (no error)"=w342, "value"=w341, "node path"=w340, "OPC UA client refnum in"=w345) -> ("error out"=w343:errorcluster, "status"=w339:u32, "OPC UA client refnum out"=w344:refnum<k21>)  [unwired: 5 in]
                        }
                        frame 109 {
                          n170 = call-poly <vilib>:"Write.vi"("error in (no error)"=w349, "value"=w348, "node path"=w347, "OPC UA client refnum in"=w352) -> ("error out"=w350:errorcluster, "status"=w346:u32, "OPC UA client refnum out"=w351:refnum<k21>)  [unwired: 5 in]
                        }
                        frame 110 {
                          n171 = call-poly <vilib>:"Write.vi"("error in (no error)"=w356, "value"=w355, "node path"=w354, "OPC UA client refnum in"=w359) -> ("error out"=w357:errorcluster, "status"=w353:u32, "OPC UA client refnum out"=w358:refnum<k21>)  [unwired: 5 in]
                        }
                        frame 111 {
                          n172 = call-poly <vilib>:"Write.vi"("error in (no error)"=w363, "value"=w362, "node path"=w361, "OPC UA client refnum in"=w366) -> ("error out"=w364:errorcluster, "status"=w360:u32, "OPC UA client refnum out"=w365:refnum<k21>)  [unwired: 5 in]
                        }
                        frame 113 {
                          n173 = To Time Stamp(1:w370) -> (0:w368:timestamp[])
                          n174 = call-poly <vilib>:"Write.vi"("error in (no error)"=w371, "value"=w368, "node path"=w369, "OPC UA client refnum in"=w374) -> ("error out"=w372:errorcluster, "status"=w367:u32, "OPC UA client refnum out"=w373:refnum<k21>)  [unwired: 5 in]
                        }
                      }
                      n175 = Set Variant Attribute(Variant=w180, name=w175, value=w179, error in=w178) -> (Variant out=w176:variant, error out=w177:errorcluster)  [unwired: 1 out]
                    }
                  }
                }
              }
              frame True {
              }
            }
            "Write Table" <- w137
            n176 = call "Global Stop Actions.vi"("Command"=Stop_Global_Commands."Read", "error in (no error)"=w134, "Stop on Error?"=FALSE, "vi reference"=w132) -> ("error out"=w128:errorcluster, "Latched Stop"=w133:bool)  [unwired: 5 in, 1 out]
            n177 = Unbundle By Name(w128) -> ("code"=→"Write Code":i32)
            n178 = call "Report Error to Process.vi"("Error"=w128, "This VI"=w129) -> ()  [unwired: 10 in]
            n179 = Wait Until Next ms Multiple(millisecond multiple=u32 1) -> ()  [unwired: 1 out]
          }
          n180 = Merge Errors(w37, w55, w38) -> (w53:errorcluster)
        }
        frame Error {
        }
      }
    }
  }
  n181 = Unbundle By Name(w7) -> ("OPC UA client Ref"=w6:refnum<k21>, "Settings.PollEngine.Settings"=w5:T4[])
  n182 = Unbundle By Name(w4) -> ("SubscriptionIDs"=w2:u32[])
  n183 = for {
    tunnel: w2 -> [w630] mode=indexing
    shift-right: [w631] -> w12
    shift-left: w6 -> [w632]
    tunnel: w5 -> [w629] mode=indexing
    tunnel: w13 -> [_]
    tunnel: [w627] -> w1 mode=indexing if=w625
    n184 = Unbundle By Name(w629) -> ("Tags"=w628:string[])
    n185 = Empty Array?(array=w628) -> (empty?=w626:bool)
    n186 = Not(x=w626) -> (.not. x?=w625:bool)
    n187 = case shown="True" w626 {
      tunnel: w632 -> [w637 w638]
      tunnel: [w636 w638] -> w631
      tunnel: w630 -> [w635 _]
      tunnel: w628 -> [w634 _]
      tunnel: [w633 _] -> w627
      frame False {
        n188 = call <vilib>:"Delete Monitored Nodes.vi"("array of node path"=w634, "subscription ID in"=w635, "OPC UA client refnum in"=w637) -> ("subscription ID out"=w633:u32, "OPC UA client refnum out"=w636:refnum<k21>)  [unwired: 5 in, 2 out]
      }
      frame True {
      }
    }
  }
  n189 = call <vilib>:"Delete Subscriptions.vi"("array of subscription ID"=w1, "OPC UA client refnum in"=w12) -> ("OPC UA client refnum out"=w18:refnum<k21>)  [unwired: 7 in, 2 out]
  n190 = call <vilib>:"Disconnect.vi"("OPC UA client refnum in"=w18) -> ("error out"=→"error out":errorcluster)  [unwired: 10 in]
